vi "RTS Parse Custom CMDs.vi"(8 "Error In":errorcluster, 9 "Array":string[](array[string]), 11 "Device Connections In":T1={"Wago ModBus Connection"=refnum, "APLUS 1 Modbus Connection"=refnum, "APLUS 2 Modbus Connection"=refnum, "APLUS 3 Modbus Connection"=refnum, "APLUS 4 Modbus Connection"=refnum, "APLUS 5 Modbus Connection"=refnum, "APLUS 6 Modbus Connection"=refnum, "APLUS 7 Modbus Connection"=refnum, "APLUS 8 Modbus Connection"=refnum, "MX 1 VISA Connection"="", "MX 2 VISA Connection"="", "MX 3 VISA Connection"="", "MX 4 VISA Connection"="", "MX 5 VISA Connection"="", "MX1"={"Base Time"=0, "Session Number"=0, "Last Data Number"={"High"=-1, "Low"=4294967295}, "Channel List"=[], "FIFO Number (0)"=0, "Channel Number (1)"=1, "Select FIFO or Channel (F:Channel)"=FALSE, "MX100 Data"={"Measurement Values out"=[], "Date/Time"=""}}, "MX2"={"Base Time"=0, "Session Number"=0, "Last Data Number"={"High"=-1, "Low"=4294967295}, "Channel List"=[], "FIFO Number (0)"=0, "Channel Number (1)"=1, "Select FIFO or Channel (F:Channel)"=FALSE, "MX100 Data"={"Measurement Values out"=[], "Date/Time"=""}}, "MX3"={"Base Time"=0, "Session Number"=0, "Last Data Number"={"High"=-1, "Low"=4294967295}, "Channel List"=[], "FIFO Number (0)"=0, "Channel Number (1)"=1, "Select FIFO or Channel (F:Channel)"=FALSE, "MX100 Data"={"Measurement Values out"=[], "Date/Time"=""}}, "MX4"={"Base Time"=0, "Session Number"=0, "Last Data Number"={"High"=-1, "Low"=4294967295}, "Channel List"=[], "FIFO Number (0)"=0, "Channel Number (1)"=1, "Select FIFO or Channel (F:Channel)"=FALSE, "MX100 Data"={"Measurement Values out"=[], "Date/Time"=""}}, "MX5"={"Base Time"=0, "Session Number"=0, "Last Data Number"={"High"=-1, "Low"=4294967295}, "Channel List"=[], "FIFO Number (0)"=0, "Channel Number (1)"=1, "Select FIFO or Channel (F:Channel)"=FALSE, "MX100 Data"={"Measurement Values out"=[], "Date/Time"=""}}} {"MX5"."Channel Number (1)" min=1 max=60 step=1; "MX5"."FIFO Number (0)" min=-1 max=2 step=1; "MX4"."Channel Number (1)" min=1 max=60 step=1; "MX4"."FIFO Number (0)" min=-1 max=2 step=1; "MX3"."Channel Number (1)" min=1 max=60 step=1; "MX3"."FIFO Number (0)" min=-1 max=2 step=1; "MX2"."Channel Number (1)" min=1 max=60 step=1; "MX2"."FIFO Number (0)" min=-1 max=2 step=1; "MX1"."Channel Number (1)" min=1 max=60 step=1; "MX1"."FIFO Number (0)" min=-1 max=2 step=1}) -> (0 "Error Out":errorcluster, 3 "Device Connections Out":T1={"Wago ModBus Connection"=refnum, "APLUS 1 Modbus Connection"=refnum, "APLUS 2 Modbus Connection"=refnum, "APLUS 3 Modbus Connection"=refnum, "APLUS 4 Modbus Connection"=refnum, "APLUS 5 Modbus Connection"=refnum, "APLUS 6 Modbus Connection"=refnum, "APLUS 7 Modbus Connection"=refnum, "APLUS 8 Modbus Connection"=refnum, "MX 1 VISA Connection"="", "MX 2 VISA Connection"="", "MX 3 VISA Connection"="", "MX 4 VISA Connection"="", "MX 5 VISA Connection"="", "MX1"={"Base Time"=0, "Session Number"=0, "Last Data Number"={"High"=-1, "Low"=4294967295}, "Channel List"=[], "FIFO Number (0)"=0, "Channel Number (1)"=1, "Select FIFO or Channel (F:Channel)"=FALSE, "MX100 Data"={"Measurement Values out"=[], "Date/Time"=""}}, "MX2"={"Base Time"=0, "Session Number"=0, "Last Data Number"={"High"=-1, "Low"=4294967295}, "Channel List"=[], "FIFO Number (0)"=0, "Channel Number (1)"=1, "Select FIFO or Channel (F:Channel)"=FALSE, "MX100 Data"={"Measurement Values out"=[], "Date/Time"=""}}, "MX3"={"Base Time"=0, "Session Number"=0, "Last Data Number"={"High"=-1, "Low"=4294967295}, "Channel List"=[], "FIFO Number (0)"=0, "Channel Number (1)"=1, "Select FIFO or Channel (F:Channel)"=FALSE, "MX100 Data"={"Measurement Values out"=[], "Date/Time"=""}}, "MX4"={"Base Time"=0, "Session Number"=0, "Last Data Number"={"High"=-1, "Low"=4294967295}, "Channel List"=[], "FIFO Number (0)"=0, "Channel Number (1)"=1, "Select FIFO or Channel (F:Channel)"=FALSE, "MX100 Data"={"Measurement Values out"=[], "Date/Time"=""}}, "MX5"={"Base Time"=0, "Session Number"=0, "Last Data Number"={"High"=-1, "Low"=4294967295}, "Channel List"=[], "FIFO Number (0)"=0, "Channel Number (1)"=1, "Select FIFO or Channel (F:Channel)"=FALSE, "MX100 Data"={"Measurement Values out"=[], "Date/Time"=""}}} {"MX5"."Channel Number (1)" min=1 max=60 step=1; "MX5"."FIFO Number (0)" min=-1 max=2 step=1; "MX4"."Channel Number (1)" min=1 max=60 step=1; "MX4"."FIFO Number (0)" min=-1 max=2 step=1; "MX3"."Channel Number (1)" min=1 max=60 step=1; "MX3"."FIFO Number (0)" min=-1 max=2 step=1; "MX2"."Channel Number (1)" min=1 max=60 step=1; "MX2"."FIFO Number (0)" min=-1 max=2 step=1; "MX1"."Channel Number (1)" min=1 max=60 step=1; "MX1"."FIFO Number (0)" min=-1 max=2 step=1})   [LabVIEW 2016]
uses:
  Type Definitions/RTS Modbus Connections.ctl
  <vilib>/NI/Modbus Library/API/Master/Modbus Master.lvclass
  Drivers/Yokogawa MX100/Type Definitions/MX100 Initialization.ctl
  Drivers/Yokogawa MX100/Type Definitions/MX100 Data.ctl
panel:
  # "ST-1,Volt-0.00,Freq-0,RstWh-1"
  # "DR-,304-0,312-0,320-0"
  # "TP-,328-90.00,329-20.00,330-65.00,331-60.00"
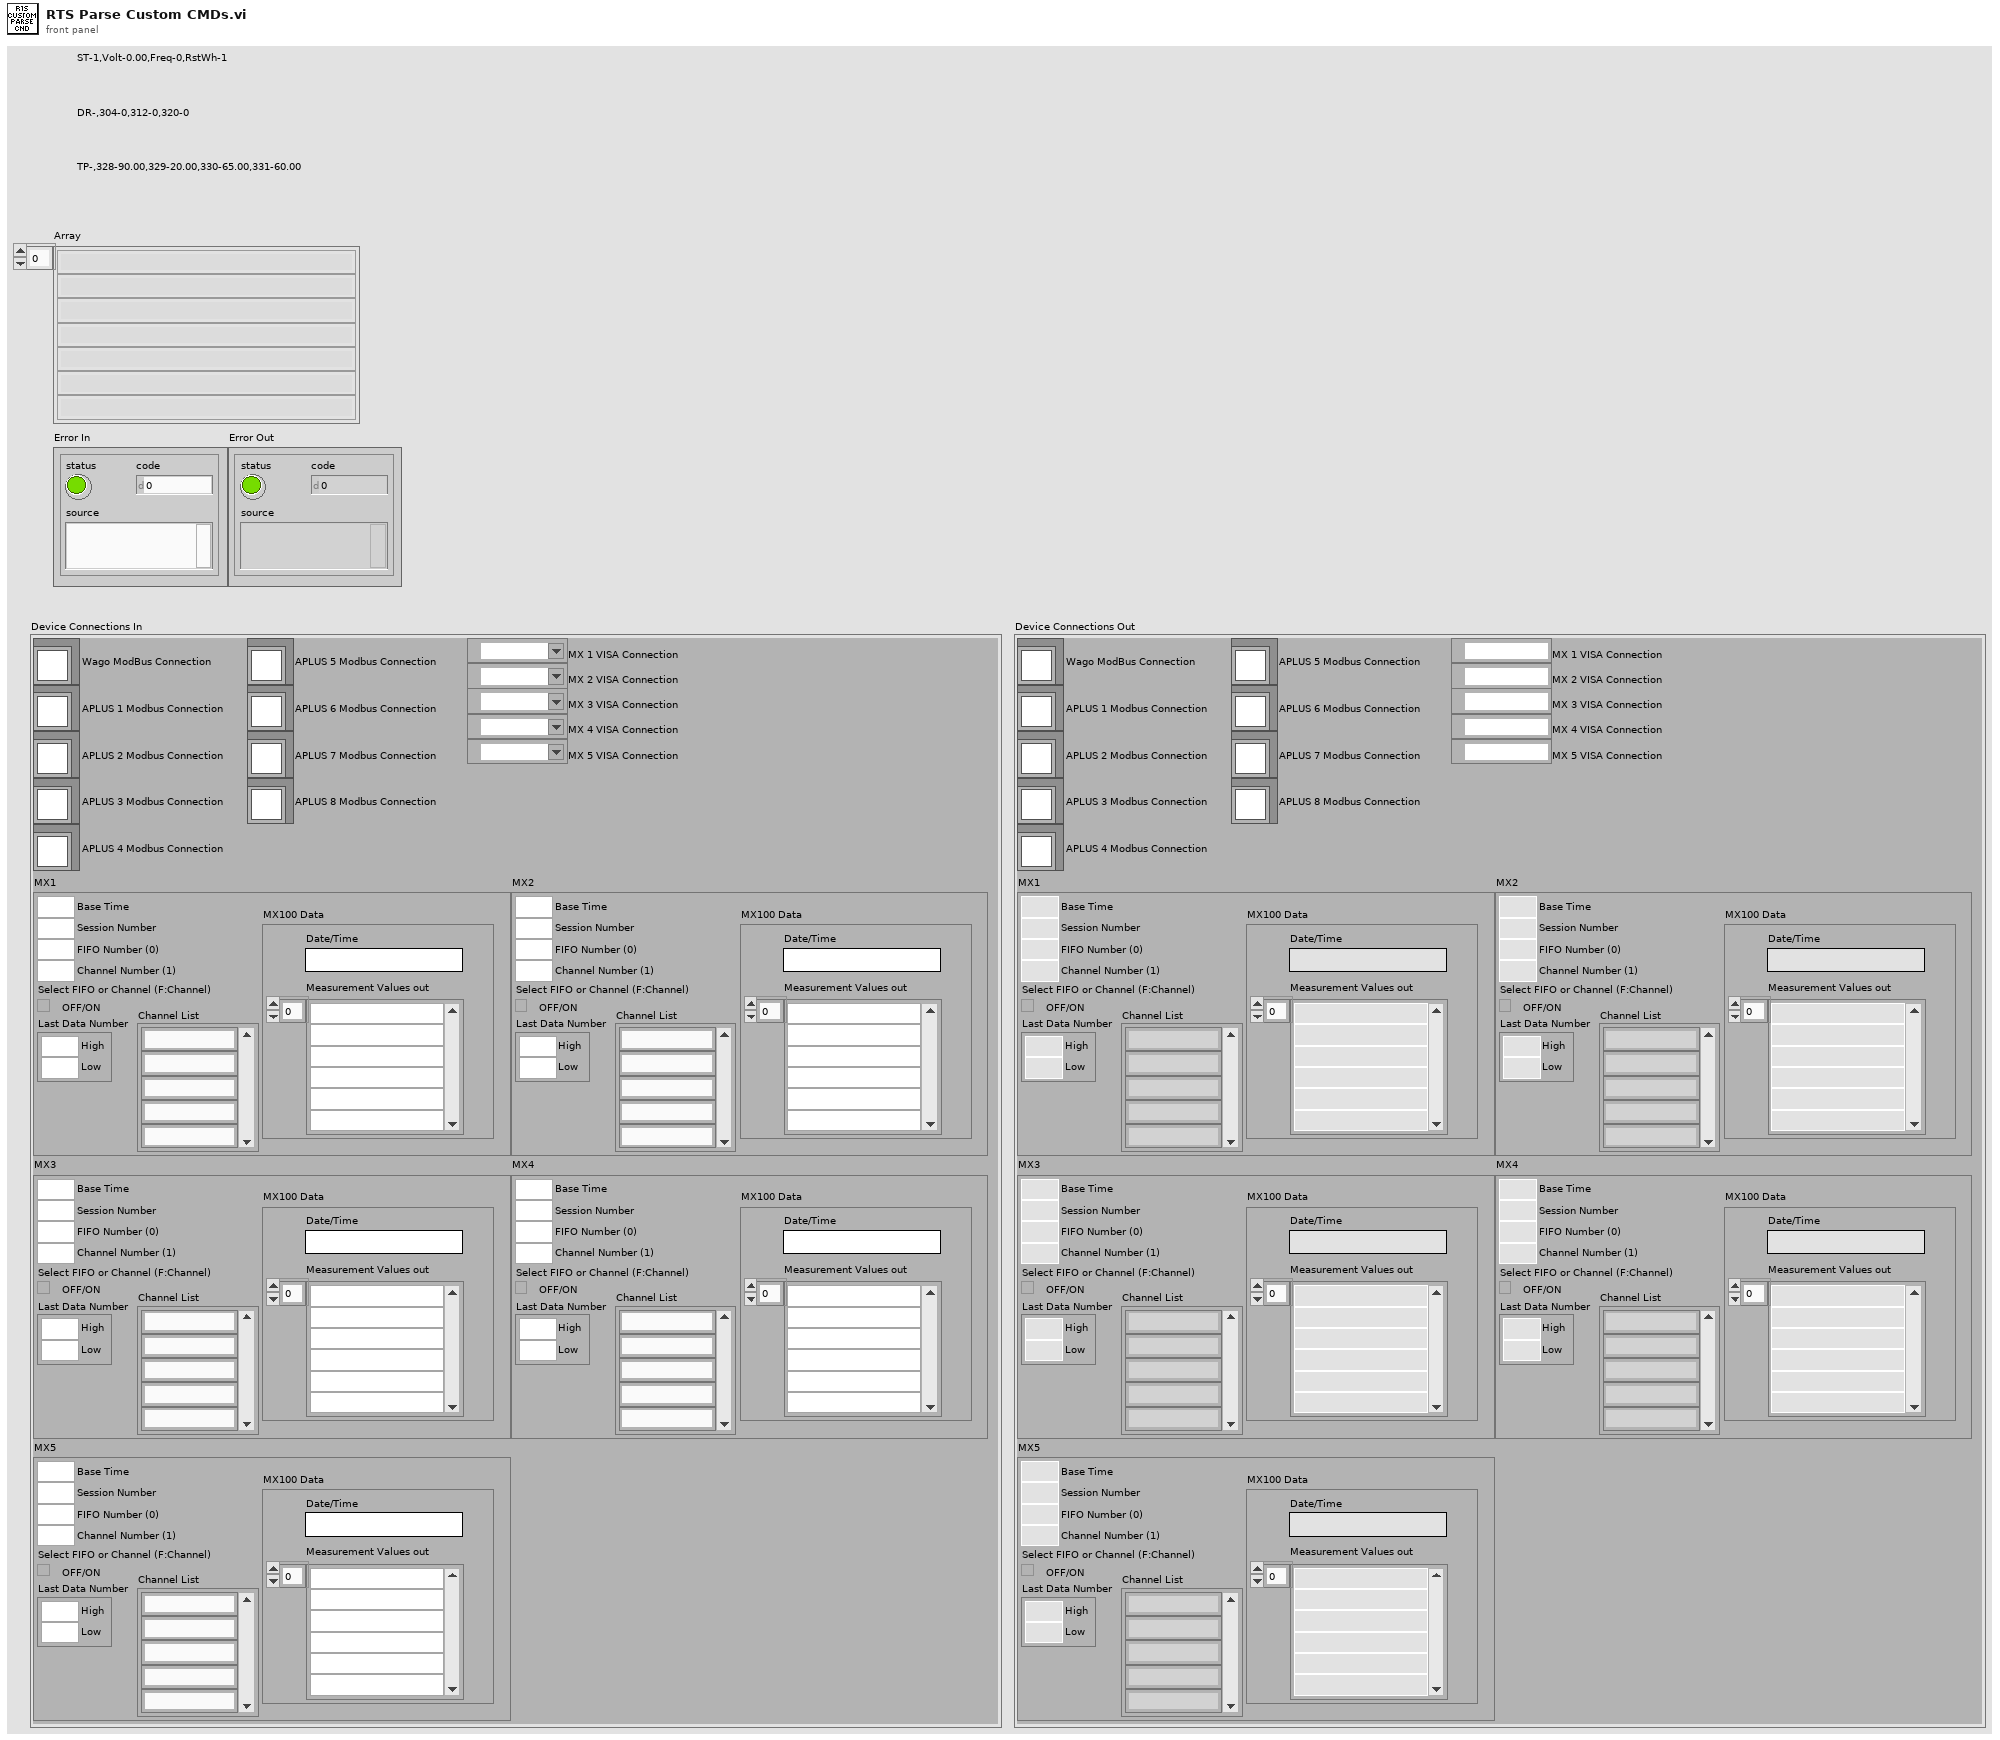
[diagram p1: front panel]
types:
  T1 = typedef "RTS Modbus Connections.ctl" = cluster{"Wago ModBus Connection":refnum<class "Modbus Master.lvclass">, "APLUS 1 Modbus Connection":refnum<class "Modbus Master.lvclass">, "APLUS 2 Modbus Connection":refnum<class "Modbus Master.lvclass">, "APLUS 3 Modbus Connection":refnum<class "Modbus Master.lvclass">, "APLUS 4 Modbus Connection":refnum<class "Modbus Master.lvclass">, "APLUS 5 Modbus Connection":refnum<class "Modbus Master.lvclass">, "APLUS 6 Modbus Connection":refnum<class "Modbus Master.lvclass">, "APLUS 7 Modbus Connection":refnum<class "Modbus Master.lvclass">, "APLUS 8 Modbus Connection":refnum<class "Modbus Master.lvclass">, "MX 1 VISA Connection":refnum<visa-resource-name>, "MX 2 VISA Connection":refnum<visa-resource-name>, "MX 3 VISA Connection":refnum<visa-resource-name>, "MX 4 VISA Connection":refnum<visa-resource-name>, "MX 5 VISA Connection":refnum<visa-resource-name>, "MX1":T2, "MX2":T2, "MX3":T2, "MX4":T2, "MX5":T2}
  T2 = typedef "MX100 Initialization.ctl" = cluster{"Base Time":i32, "Session Number":i32, "Last Data Number":cluster{"High":i32, "Low":u32}, "Channel List":string[], "FIFO Number (0)":i32, "Channel Number (1)":i32, "Select FIFO or Channel (F:Channel)":bool, "MX100 Data":T3}
  T3 = typedef "MX100 Data.ctl" = cluster{"Measurement Values out":dbl[], "Date/Time":string}
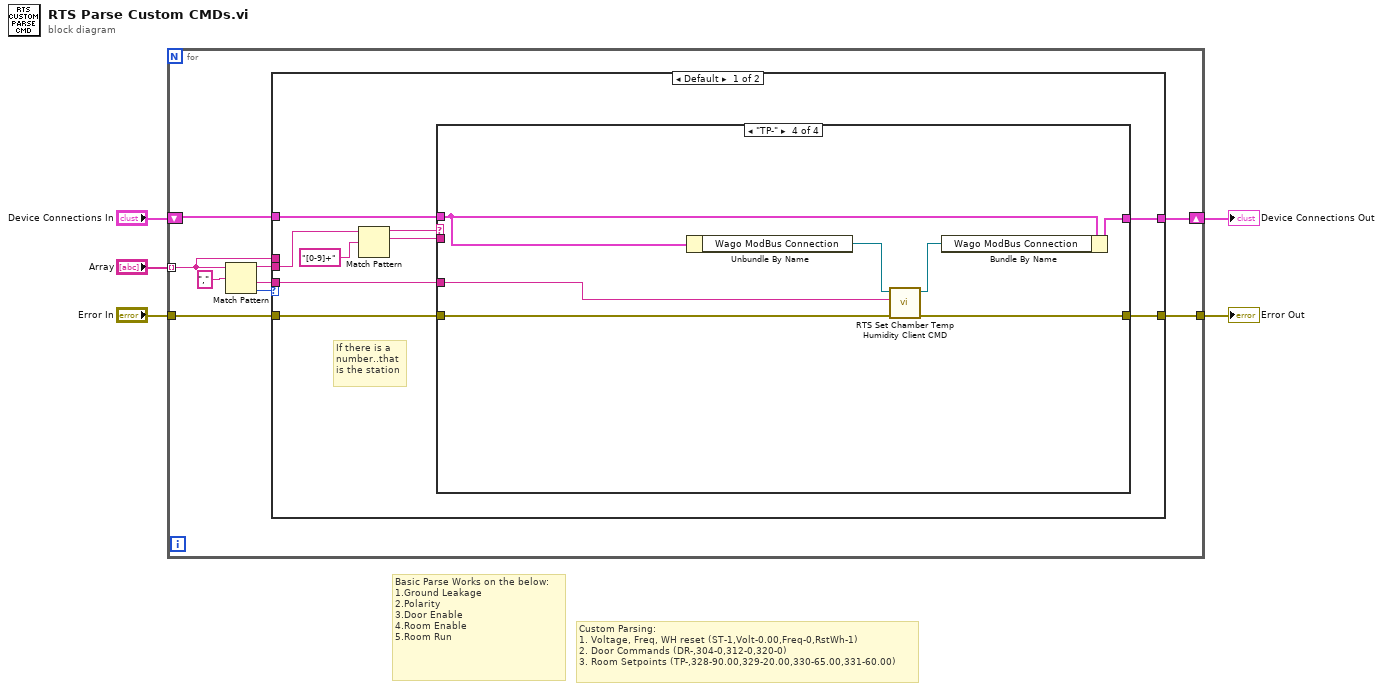
[diagram p0: block diagram]
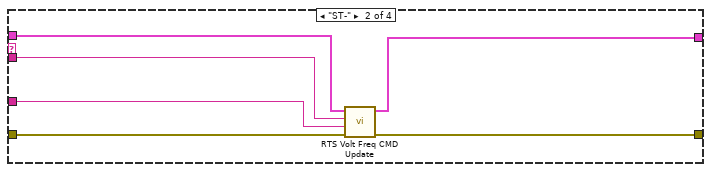
[diagram p3: hidden frame]
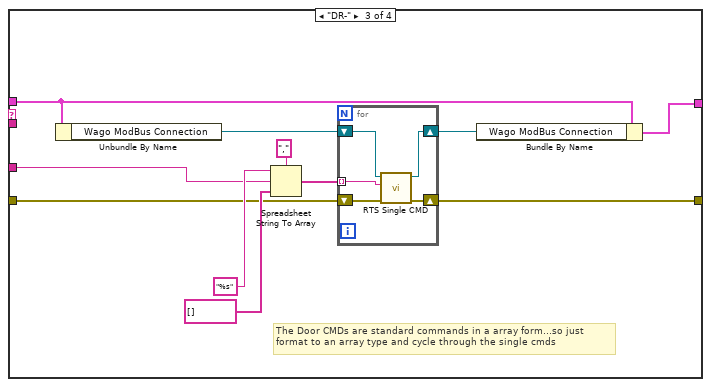
[diagram p4: hidden frame]
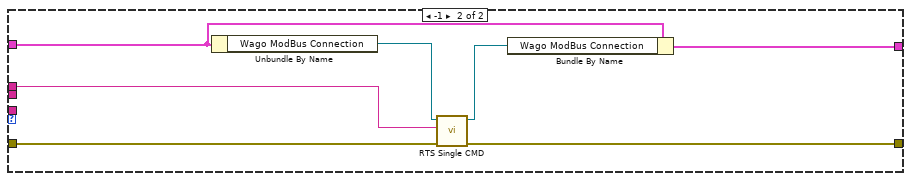
[diagram p5: hidden frame]
diagram:
  # "Custom Parsing:\n1. Voltage, Freq, WH reset (ST-1,Volt-0.00,Freq-0,RstWh-1)\n2. Door Commands (DR-,304-0,312-0,320-0)\n3. Room Setpoints (TP-,328-90.00,329-20.00,330-65.00,331-60.00)"
  # "Basic Parse Works on the below:\n1.Ground Leakage\n2.Polarity\n3.Door Enable\n4.Room Enable\n5.Room Run"
  n1 = for {
    tunnel: "Error In" -> [w13]
    tunnel: [w14] -> w4
    tunnel: "Array" -> [w12] mode=indexing
    shift-right: [w6] -> w1
    shift-left: "Device Connections In" -> [w7]
    n2 = Match Pattern(string=w12, regular expression=",") -> (before substring=w9:string, after substring=w8:string, offset past match=w10:i32)  [unwired: 1 in, 1 out]
    n3 = case shown="Default" w10 {
      tunnel: [w21 w61] -> w14
      tunnel: w13 -> [w22 w60]
      tunnel: w12 -> [_ w59]
      tunnel: w9 -> [w17 _]
      tunnel: w8 -> [w23 _]
      tunnel: w7 -> [w20 w57]
      tunnel: [w19 w55] -> w6
      frame Default {
        # "If there is a \nnumber..that\nis the station"
        n4 = Match Pattern(string=w17, regular expression="[0-9]+") -> (before substring=w16:string, match substring=w15:string)  [unwired: 1 in, 2 out]
        n5 = case shown="\"TP-\"" w16 {
          tunnel: w23 -> [_ w29 w39 w52]
          tunnel: w22 -> [w24 w28 w37 w54]
          tunnel: [w24 w27 w36 w53] -> w21
          tunnel: w20 -> [w25 w31 w34 w50]
          tunnel: [w25 w26 w32 w49] -> w19
          tunnel: w15 -> [_ w30 _ _]
          frame Default {
          }
          frame "ST-" {
            n6 = call "RTS Volt Freq CMD Update.vi"("Error In"=w28, "Data String"=w29, "Station Number"=w30, "Device Connections In"=w31) -> ("Error Out"=w27:errorcluster, "Device Connections Out"=w26:T1)  [unwired: 6 in]
          }
          frame "DR-" {
            # "The Door CMDs are standard commands in a array form...so just\nformat to an array type and cycle through the single cmds"
            n7 = Unbundle By Name(w34) -> ("Wago ModBus Connection"=w35:refnum<class "Modbus Master.lvclass">)
            n8 = Spreadsheet String To Array(delimiter (Tab)=",", format string="%s", spreadsheet string=w39, array type (2D Dbl)=string[] []) -> (array=w38:string[])
            n9 = for {
              tunnel: w38 -> [w47] mode=indexing
              shift-right: [w45] -> w36
              shift-left: w37 -> [w46]
              shift-right: [w43] -> w33
              shift-left: w35 -> [w44]
              n10 = call "RTS Single CMD.vi"("error in (no error)"=w46, "String"=w47, "Modbus Master in"=w44) -> ("error out"=w45:errorcluster, "Modbus Master out"=w43:refnum<class "Modbus Master.lvclass">)  [unwired: 7 in]
            }
            n11 = Bundle By Name(cluster=w34, "Wago ModBus Connection"=w33) -> (w32:T1)
          }
          frame "TP-" {
            n12 = Unbundle By Name(w50) -> ("Wago ModBus Connection"=w51:refnum<class "Modbus Master.lvclass">)
            n13 = call "RTS Set Chamber Temp Humidity Client CMD.vi"("error in (no error)"=w54, "Data String"=w52, "Modbus Master in"=w51) -> ("error out"=w53:errorcluster, "Modbus Master Out"=w48:refnum<class "Modbus Master.lvclass">)  [unwired: 7 in]
            n14 = Bundle By Name(cluster=w50, "Wago ModBus Connection"=w48) -> (w49:T1)
          }
        }
      }
      frame -1 {
        n15 = Unbundle By Name(w57) -> ("Wago ModBus Connection"=w58:refnum<class "Modbus Master.lvclass">)
        n16 = call "RTS Single CMD.vi"("error in (no error)"=w60, "String"=w59, "Modbus Master in"=w58) -> ("error out"=w61:errorcluster, "Modbus Master out"=w56:refnum<class "Modbus Master.lvclass">)  [unwired: 7 in]
        n17 = Bundle By Name(cluster=w57, "Wago ModBus Connection"=w56) -> (w55:T1)
      }
    }
  }
  "Error Out" <- w4
  "Device Connections Out" <- w1
